vi "Data Access.vi"(8 "error in (no error)":errorcluster, 10 "Data Access Handler":refnum<class "Data Access Handler.lvclass">, 11 "DMM List Triggers Msg in":refnum<class "DMM List Triggers Msg.lvclass">) -> (0 "error out":errorcluster, 3 "DMM List Triggers Msg out":refnum<class "DMM List Triggers Msg.lvclass">)   [LabVIEW 2020, in "DMM Msg.lvlib" / "DMM List Triggers Msg.lvclass"]
doc: "Expose class private data to the front panel while letting the Data Access Handler class act on the data."
uses:
  DMM List Triggers Msg.lvclass
  C:/Current projects/WS/PPL/HDH.Actor Framework.Core.Msg.lvlibp/Flex Msg/Flex Msg.lvclass
  PPL/HDH.Actor Framework.Core.Msg.lvlibp/Flex Msg/Data Access Handlers/Data Access Handler/Data Access Handler.lvclass
  PPL/HDH.Actor Framework.Core.Publisher.lvlibp/Messages/Response Msg/Response Core/Controls/Ctl_SendFunction.ctl
  PPL/HDH.Actor Framework.Core.Instrument Handler.lvlibp/Messages/Instrument Msg/Instrument Msg.lvclass
  C:/Current projects/WS/PPL/HDH.Actor Framework.Core.Instrument Handler.lvlibp/Messages/Instrument Msg/Instrument Msg.lvclass
  PPL/HDH.Actor Framework.Core.Publisher.lvlibp
panel:
  in  "Message Priority":enum16{"Low", "Normal", "High"}(ring)=enum."Normal"
  in  "Timeout if Waiting":i32=-1
  in  "Send Function":T1=enum."Await Reply"
  in  "Cancel":bool
  in  "OK":bool
  # "Send details"
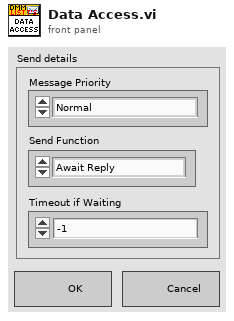
[diagram p1: front panel]
types:
  T1 = typedef "HDH.Actor Framework.Core.Publisher.lvlibp/Ctl_SendFunction.ctl" = enum16{"Send and Forget", "Request Reply", "Await Reply"}
  T2 = typedef "HDH.Actor Framework.Core.Actor.lvlibp/Message Enqueuer.lvclass/Message Priority.ctl" = enum16{"Low", "Normal", "High"}
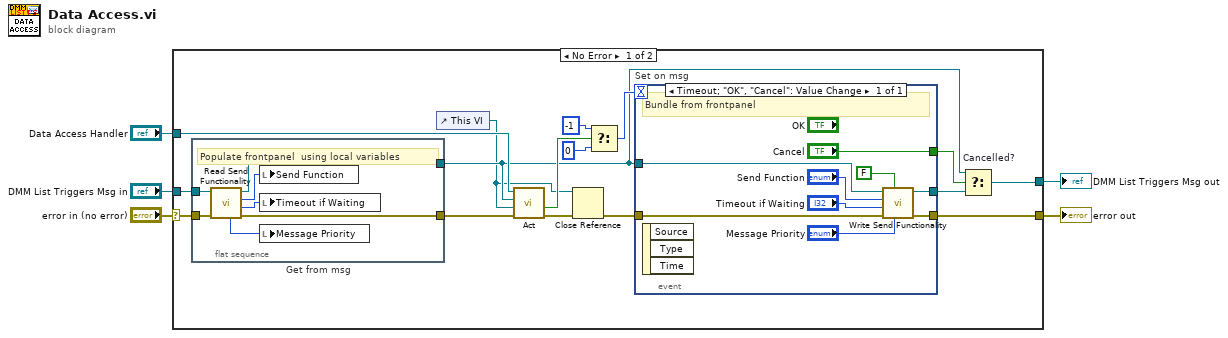
[diagram p0: block diagram]
diagram:
  n1 = case shown="No Error" "error in (no error)" {
    selector: "error in (no error)" -> [w21 w39]
    tunnel: [w14 w39] -> w4
    tunnel: [w9 w38] -> w2
    tunnel: "DMM List Triggers Msg in" -> [w12 w38]
    tunnel: "Data Access Handler" -> [w20 _]
    frame No Error {
      n2 = flat-sequence "Get from msg" {
        tunnel: w21 -> [w36]
        tunnel: [w34] -> w7
        tunnel: w12 -> [w37]
        tunnel: [w35] -> w19
        frame #0 {
          # "Populate frontpanel  using local variables"
          n3 = call "Read Send Functionality.vi"("error in (no error)"=w36, "Instrument Msg in"=w37) -> ("error out"=w35:errorcluster, "Timeout if Waiting"=w32:i32, "Send Function"=w33:T1, "Instrument Msg out"=w34:refnum<class "DMM List Triggers Msg.lvclass">, "Message Priority"=w31:T2)  [unwired: 4 in, 1 out]
          n4 = local write "Send Function"(w33) -> ()
          n5 = local write "Timeout if Waiting"(w32) -> ()
          n6 = local write "Message Priority"(w31) -> ()
        }
      }
      n7 = control-ref of="This VI"() -> (w6:refnum<vi>)
      n8 = call-dynamic "Act.vi"("error in (no error)"=w19, "VI Refnum in"=w6, "Flex Msg type"=w7, "Data Access Handler in"=w20) -> ("error out"=w11:errorcluster, "Await user action?"=w18:bool)  [unwired: 5 in, 1 out]
      n9 = Close Reference(reference=w6, error in (no error)=w11) -> (error out=w13:errorcluster)
      n10 = Select(t=-1, s=w18, f=0 ("t")) -> (s? t:f=w15:i32)
      n11 = event "Set on msg" shown="[0] Timeout;  \"OK\", \"Cancel\": Value Change" {
        selector: _ -> [_]
        dyn-events: _ -> [_]
        timeout: w15 -> [_]
        tunnel: [w26] -> w14
        tunnel: w13 -> [w27]
        tunnel: ["Cancel"] -> w10
        tunnel: [w28] -> w8
        tunnel: w7 -> [w29]
        event Timeout; "OK", "Cancel": Value Change {
          # "Bundle from frontpanel"
          n12 = event-data() -> ()  [unwired: 1 in, 3 out]
          n13 = call "Write Send Functionality.vi"("Message Priority(Normal)"="Message Priority", "Publish Data?(T)"=FALSE, "error in (no error)"=w27, "Timeout if Waiting(-1ms)"="Timeout if Waiting", "Send Function(Await Reply)"="Send Function", "Instrument Msg in"=w29) -> ("error out"=w26:errorcluster, "Instrument Msg out"=w28:refnum<class "DMM List Triggers Msg.lvclass">)  [unwired: 4 in]
        }
      }
      n14 = Select "Cancelled?"(t=w7, s=w10, f=w8) -> (s? t:f=w9:refnum<class "DMM List Triggers Msg.lvclass">)
    }
    frame Error {
    }
  }
  "error out" <- w4
  "DMM List Triggers Msg out" <- w2
